vi "Send routine test.vi"() -> ()   [LabVIEW 2018]
panel:
  in  "stop":bool
  in  "?":bool
  out "ERROR":bool
  out "OK":bool
  out "Responses":string[](array[string])
  out "error out":errorcluster
  in  "instructions":string[](array[string])=["STOP", "SR0=0"]
  in  "port":string
  in  "ip":string
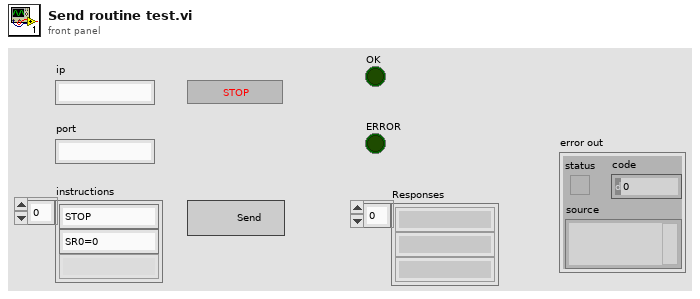
[diagram p1: front panel]
types:
  T1 = enum16{"Standard", "Buffered", "CRLF", "Immediate"}
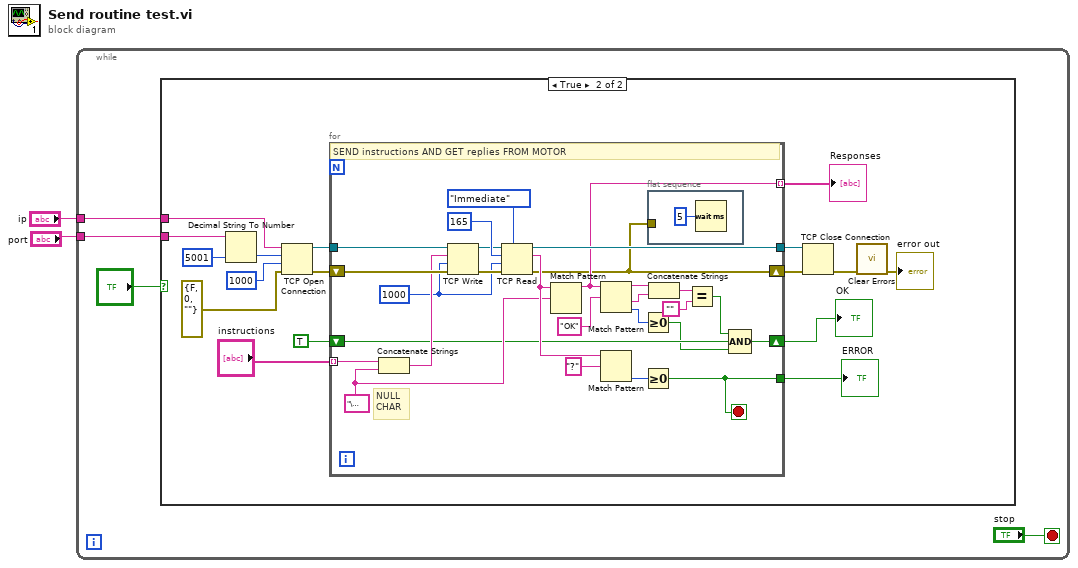
[diagram p0: block diagram]
diagram:
  n1 = while {
    tunnel: "ip" -> [w6]
    tunnel: "port" -> [w5]
    stop <- "stop" stop-if-true
    n2 = case shown="True" "?" {
      tunnel: w6 -> [_ w11]
      tunnel: w5 -> [_ w10]
      frame False {
      }
      frame True {
        n3 = Decimal String To Number(string=w10, default (0L)=u16 5001 ("default (0 I32)")) -> (number=w21:u16)  [unwired: 1 in, 1 out]
        n4 = TCP Open Connection(address=w11, remote port or service name=w21, timeout ms (60000)=1000, error in (no error)=errorcluster {"status"=FALSE, "code"=0, "source"=""}) -> (connection ID=w19:refnum<k5>, error out=w20:errorcluster)  [unwired: 1 in]
        n5 = for {
          tunnel: "instructions" -> [w50] mode=indexing
          tunnel: w19 -> [w44]
          tunnel: [w33] -> w18
          shift-right: [w29] -> w14
          shift-left: TRUE -> [w28]
          tunnel: [w26] -> w16
          shift-right: [w24] -> w15
          shift-left: w20 -> [w46]
          tunnel: [w25] -> w13 mode=indexing
          stop <- w33 stop-if-true
          w42 = 1000 ("timeout ms (60000)")
          w32 = "\u0000" ("search string")
          # "NULL\nCHAR"
          # "SEND instructions AND GET replies FROM MOTOR"
          n6 = Concatenate Strings(w50, w32) -> (w43:string)
          n7 = TCP Write(connection ID=w44, data in=w43, error in (no error)=w46, 9:w42) -> (connection ID out=w47:refnum<k5>, error out=w49:errorcluster)  [unwired: 1 out]
          n8 = TCP Read(connection ID=w47, bytes to read=165, error in (no error)=w49, 7:T1."Immediate" ("mode (standard)"), 9:w42) -> (connection ID out=w26:refnum<k5>, data out=w34:string, error out=w24:errorcluster)
          n9 = Match Pattern(string=w34, regular expression=w32) -> (before substring=w25:string)  [unwired: 1 in, 3 out]
          n10 = Match Pattern(string=w25, regular expression="OK" ("y")) -> (before substring=w36:string, after substring=w39:string, offset past match=w31:i32)  [unwired: 1 in, 1 out]
          n11 = Match Pattern(string=w34, regular expression="?") -> (offset past match=w41:i32)  [unwired: 1 in, 3 out]
          n12 = Greater Or Equal To 0?(x=w31) -> (x >= 0?=w27:bool)
          n13 = Greater Or Equal To 0?(x=w41) -> (x >= 0?=w33:bool)
          n14 = flat-sequence {
            tunnel: w24 -> [_]
            frame #0 {
              n15 = Wait (ms)(milliseconds to wait=u32 5) -> ()  [unwired: 1 out]
            }
          }
          n16 = Concatenate Strings(w36, w39) -> (w37:string)
          n17 = Equal?(x=w37, y="") -> (x = y?=w30:bool)
          n18 = Compound Arithmetic op=AND(w30, w28, w27) -> (w29:bool)
        }
        "Responses" <- w13
        "OK" <- w14
        "ERROR" <- w18
        n19 = TCP Close Connection(connection ID=w16, error in (no error)=w15) -> (error out=w12:errorcluster)  [unwired: 1 in, 1 out]
        n20 = call <vilib>:"Clear Errors.vi"("error in (no error)"=w12) -> ("error out"=→"error out":errorcluster)  [unwired: 5 in, 1 out]
      }
    }
  }
